vi "Stop Core.vi"(10 "final error code":i32, 11 "ClientUI in":refnum<class "ClientUI.lvclass">) -> (3 "ClientUI out":refnum<class "ClientUI.lvclass">)   [LabVIEW 2018, in "ClientUI.lvlib" / "ClientUI.lvclass"]
doc: "(<B>Filename</B>: Actor Framework.lvlib:Actor.lvclass:Stop Core.vi)\n\nDefines what the actor does before it stops. Use the <B>final error code</B> input to determine whether the actor shut down in response to an error.\n\nBy default, this method passes the Stop message along to all auto-stop nested actors. A descendant class may override this method to define additional behavior, such as shutting down any processes the actor initiated in its override of the Actor Core method."
uses:
  ClientUI.lvclass
  <vilib>/ActorFramework/Time-Delayed Send Message/Time-Delay Override Options.ctl
  ClientUI.lvclass/ClientUI.ctl
  TCP_Client/TCP_Client/TCP_Client.lvclass
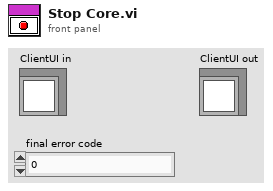
[diagram p1: front panel]
types:
  T1 = typedef "Time-Delay Override Options.ctl" = enum16{"Send next copy now", "Skip next scheduled copy", "Send next copy now and stop all further copies", "Stop all further copies"}
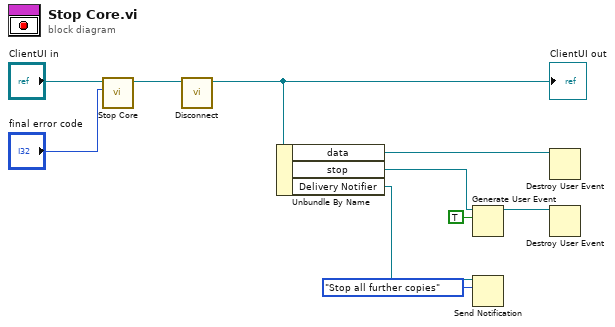
[diagram p0: block diagram]
diagram:
  n1 = call-parent "Stop Core.vi"("final error code"="final error code", "Actor in"="ClientUI in") -> ("Actor out"=w2:refnum<class "ClientUI.lvclass">)  [unwired: 9 in]
  n2 = call-dynamic "Disconnect.vi"("TCP_Client in"=w2) -> ("TCP_Client out"=w1:refnum<class "ClientUI.lvclass">)  [unwired: 9 in, 1 out]
  "ClientUI out" <- w1
  n3 = Unbundle By Name(w1) -> ("data"=w8:refnum<user-event>, "stop"=w7:refnum<user-event>, "Delivery Notifier"=w4:refnum<notifier>)
  n4 = Generate User Event(user event=w7, event data cluster=TRUE ("event data")) -> (user event out=w5:refnum<user-event>)  [unwired: 2 in, 1 out]
  n5 = Send Notification(notification=Time-Delay_Override_Options."Stop all further copies", notifier=w4) -> ()  [unwired: 1 in, 2 out]
  n6 = Destroy User Event(user event=w8) -> ()  [unwired: 1 in, 1 out]
  n7 = Destroy User Event(user event=w5) -> ()  [unwired: 1 in, 1 out]
